vi "Manual print UI.vi"() -> (0 "Print?":bool, 1 "ECU Info":T2, 2 "Parttype":T1, 3 "SN":string)   [LabVIEW 2018]
uses:
  typedefs/parttype.ctl
panel:
  in  "Cancel":bool
  in  "Print":bool
  in  "Parttype":T1
  in  "SN":string
  in  "ECU Info":T2
  # "Manual Print"
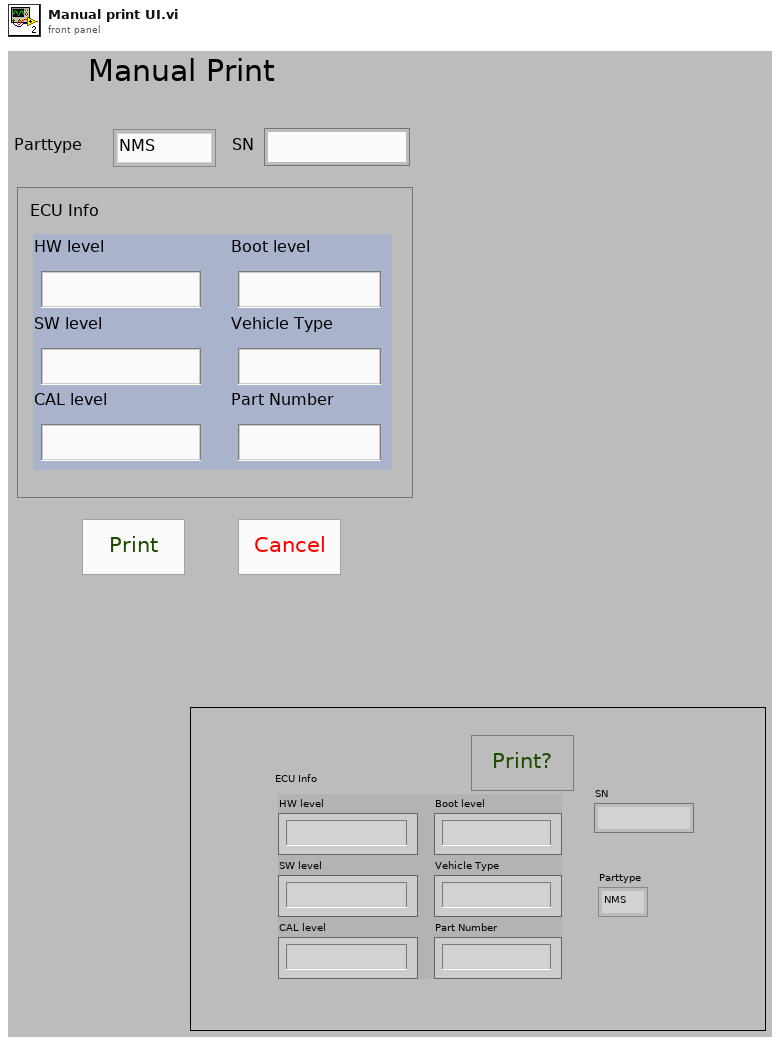
[diagram p1: front panel]
types:
  T1 = typedef "parttype.ctl" = enum16{"NMS", "B-SUV"}
  T2 = cluster{"HW level":string, "SW level":string, "CAL level":string, "Boot level":string, "Vehicle Type":string, "Part Number":string}
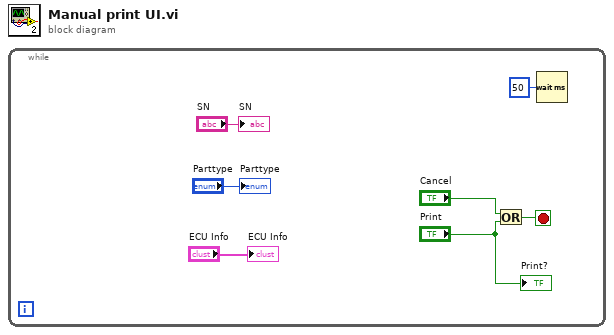
[diagram p0: block diagram]
diagram:
  n1 = while {
    stop <- w3 stop-if-true
    n2 = Or(x="Cancel", y="Print") -> (x .or. y?=w3:bool)
    n3 = Wait (ms)(milliseconds to wait=u32 50) -> ()  [unwired: 1 out]
    "SN" <- "SN"
    "ECU Info" <- "ECU Info"
    "Print?" <- "Print"
    "Parttype" <- "Parttype"
  }
